vi "DAQ.GetPublicEvents.vi"(8 "error in (no error)":errorcluster, 11 "DAQ":refnum<class "DAQ.lvclass">) -> (0 "error out":errorcluster, 2 "Public Events":T1, 3 "DAQ out":refnum<class "DAQ.lvclass">)   [LabVIEW 2016, in "DAQ.lvclass"]
doc: "---------------------------------------------------------------\nJKI State Machine Objects™\nhttp://jki.net/state-machine-objects/\nCopyright (C) 2005-2015, JKI <info@jki.net>\nALL RIGHTS RESERVEDJKI State Machine Objects (SMO) 1.0.0.4\nJKI - JKI\nCopyright (c) 2015, JKI"
uses:
  DAQ.lvclass
  Typedefs/PublicEvents--Cluster.ctl
  Typedefs/PublicEvents--DAQ.Read.ctl
  Typedefs/PublicEvents--DAQ.Write.ctl
  DAQ.lvclass/DAQ.ctl
panel:
  # "For instructions on how to use the JKI State Machine Objects, examples and video tutorials, visit:\nhttp://jki.net/state-machine-objects/\n\nJKI State Machine Objects™\nhttp://jki.net/state-machine-objects/\nCopyright (C) 2005-2015, JKI <info@jki.net>\nALL RIGHTS RESERVED"
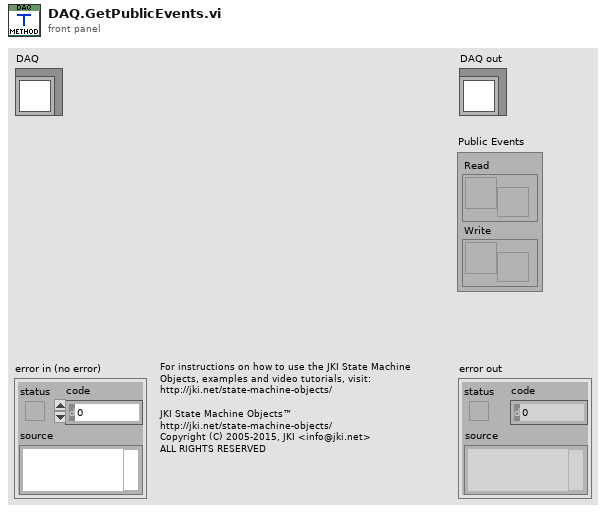
[diagram p1: front panel]
types:
  T1 = typedef "DAQ.lvclass/PublicEvents--Cluster.ctl" = cluster{"Read":refnum<user-event>, "Write":refnum<user-event>}
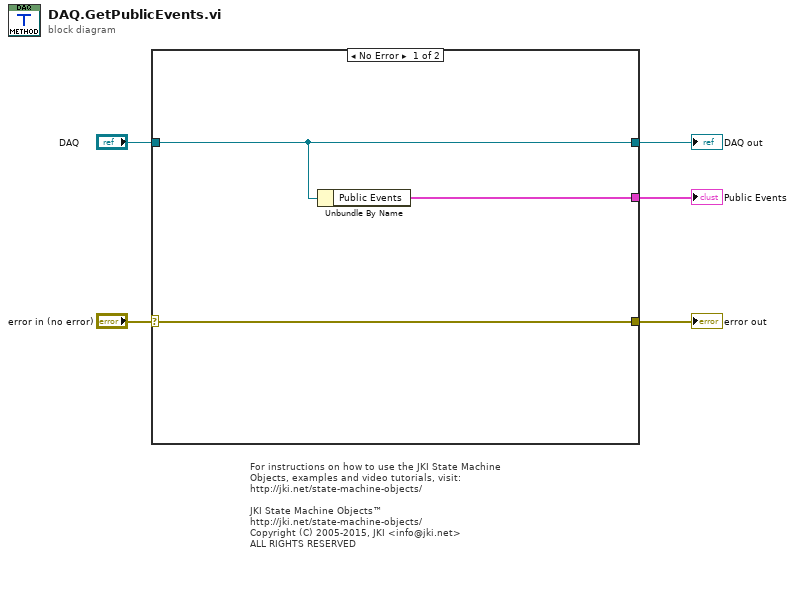
[diagram p0: block diagram]
diagram:
  # "For instructions on how to use the JKI State Machine Objects, examples and video tutorials, visit:\nhttp://jki.net/state-machine-objects/\n\nJKI State Machine Objects™\nhttp://jki.net/state-machine-objects/\nCopyright (C) 2005-2015, JKI <info@jki.net>\nALL RIGHTS RESERVED"
  n1 = case shown="No Error" "error in (no error)" {
    selector: "error in (no error)" -> [w7 w9]
    tunnel: "DAQ" -> [w6 w10]
    tunnel: [w7 w9] -> w4
    tunnel: [w6 w10] -> w3
    tunnel: [w8 _] -> w1
    frame No Error {
      n2 = Unbundle By Name(w6) -> ("Public Events"=w8:T1)
    }
    frame Error {
    }
  }
  "error out" <- w4
  "DAQ out" <- w3
  "Public Events" <- w1
